vi "intensity gate sort.vi"(6 "Y array in":dbl[](array[numeric]), 8 "error in (no error)":errorcluster, 9 "Energy 2d gate":T1, 10 "which spectrum":string, 11 "X array in":dbl[](array[numeric])) -> (0 "error out (no error)":errorcluster, 4 "Intensity plot":u64[][](array[numeric]))   [LabVIEW 2016]
uses:
  controls/energy 2d selection.ctl
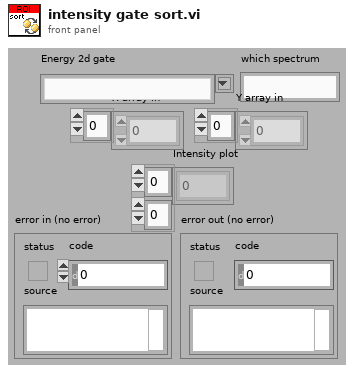
[diagram p1: front panel]
types:
  T1 = typedef "energy 2d selection.ctl" = string
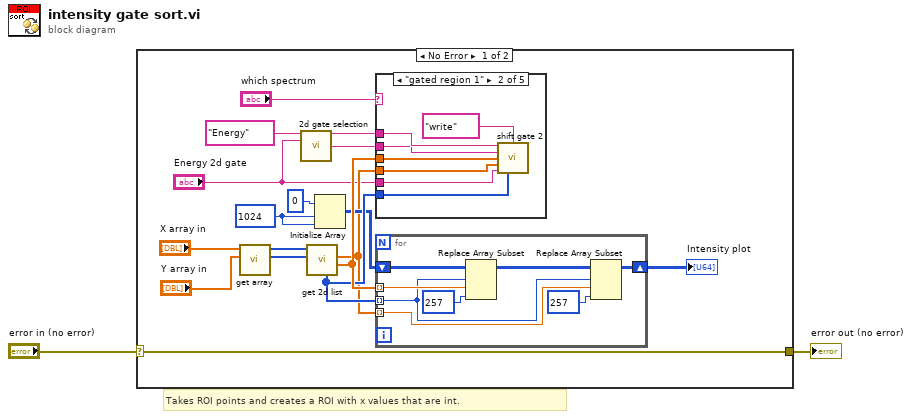
[diagram p0: block diagram]
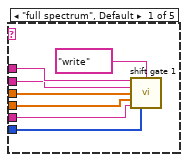
[diagram p2: hidden frame]
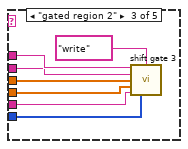
[diagram p3: hidden frame]
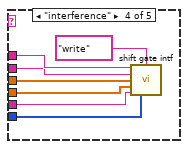
[diagram p4: hidden frame]
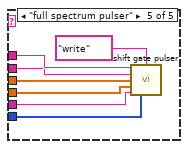
[diagram p5: hidden frame]
diagram:
  # "Takes ROI points and creates a ROI with x values that are int."
  n1 = case shown="No Error" "error in (no error)" {
    selector: "error in (no error)" -> [w3 w63]
    tunnel: [w3 w63] -> w1
    frame No Error {
      w13 = 1024 ("dimension size")
      n2 = call "get array.vi"("y array in"="Y array in", "x array in"="X array in") -> ("y out array"=w8:i32[], "x out array"=w7:i32[])  [unwired: 7 in, 1 out]
      n3 = call "2d gate selection.vi"("time or energy"="Energy", "Energy 2d gate"="Energy 2d gate") -> ("Y name"=w10:string, "X name"=w11:string)  [unwired: 7 in, 5 out]
      n4 = call "get 2d list.vi"("Y"=w8, "X"=w7) -> ("upper limit"=w16:dbl[], "lower limit"=w5:dbl[], "X Values"=w15:u32[])  [unwired: 6 in, 1 out]
      n5 = Initialize Array(u64 0 ("element"), w13, w13) -> (w14:u64[][])
      n6 = case shown="\"gated region 1\"" "which spectrum" {
        tunnel: w15 -> [w33 w40 w47 w54 w61]
        tunnel: w16 -> [w32 w39 w46 w53 w60]
        tunnel: w5 -> [w31 w38 w45 w52 w59]
        tunnel: w10 -> [w30 w37 w44 w51 w58]
        tunnel: w11 -> [w29 w36 w43 w50 w57]
        tunnel: "Energy 2d gate" -> [w28 w35 w42 w49 w56]
        frame "full spectrum", Default {
          n7 = call "shift gate 1.vi"("X name"=w30, "shift control"="write", "Y name"=w29, "Y range"=w32, "Y range Min"=w31, "Energy 2d gate in"=w28, "X range"=w33) -> ()  [unwired: 2 in, 7 out]
        }
        frame "gated region 1" {
          n8 = call "shift gate 2.vi"("X name"=w37, "shift control"="write", "Y name"=w36, "Y range max"=w39, "Y range Min"=w38, "Energy 2d gate in"=w35, "X range"=w40) -> ()  [unwired: 2 in, 7 out]
        }
        frame "gated region 2" {
          n9 = call "shift gate 3.vi"("X name"=w44, "shift control"="write", "Y name"=w43, "Y range max"=w46, "Y range Min"=w45, "Energy 2d gate in"=w42, "X range"=w47) -> ()  [unwired: 2 in, 7 out]
        }
        frame "interference" {
          n10 = call "shift gate intf.vi"("X name"=w51, "shift control"="write", "Y name"=w50, "Y range max"=w53, "Y range Min"=w52, "Energy 2d gate in"=w49, "X range"=w54) -> ()  [unwired: 2 in, 7 out]
        }
        frame "full spectrum pulser" {
          n11 = call "shift gate pulser.vi"("X name"=w58, "shift control"="write", "Y name"=w57, "Y range"=w60, "Y range Min"=w59, "Energy 2d gate in"=w56, "X range"=w61) -> ()  [unwired: 2 in, 7 out]
        }
      }
      n12 = for {
        tunnel: w16 -> [w26] mode=indexing
        tunnel: w15 -> [w23] mode=indexing
        tunnel: w5 -> [w22] mode=indexing
        shift-right: [w20] -> w17
        shift-left: w14 -> [w27]
        n13 = Replace Array Subset(array=w27, new element=257 ("new element/subarray"), index (row)=w23, index (col)=w26) -> (w24:u64[][])
        n14 = Replace Array Subset(array=w24, new element=257 ("new element/subarray"), index (row)=w23, index (col)=w22) -> (w20:u64[][])
      }
      "Intensity plot" <- w17
    }
    frame Error {
    }
  }
  "error out (no error)" <- w1
